vi "PH_ImageCoG_Plotter.Reset.vi"(0 "i ref in":refnum<vi>, 5 "error in":errorcluster) -> (14 "i ref out":refnum<vi>, 19 "error out":errorcluster)   [LabVIEW 2014, in "PH_ImageCoG_Plotter.lvlib"]
doc: "This VI resets some GUI elements and some attributes."
uses:
  PH_ImageCoG_Plotter.lvlib
  <vilib>/vision/Image Controls.llb/IMAQ Image.ctl
  PH_Common/PH_Common.lvlib
  PH_Img_BaseClass/PH_Img_BaseClass.lvlib
panel:
  in  "Image":T1
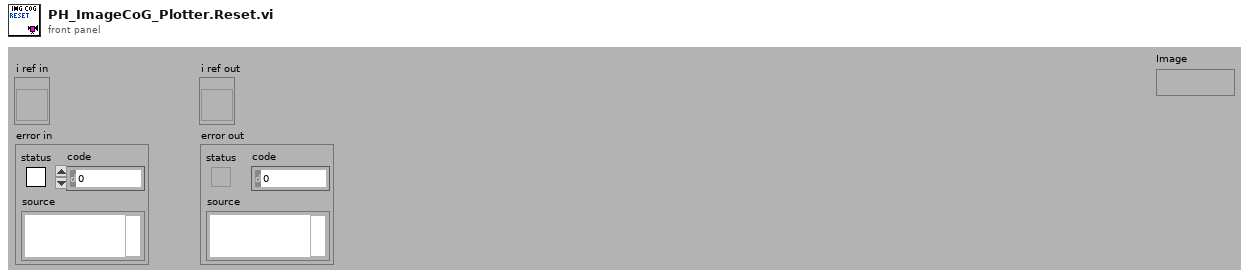
[diagram p1: front panel]
types:
  T1 = typedef "IMAQ Image.ctl" = refnum<image>
  T2 = typedef "PH_ImageCoG_Plotter.lvlib/PH_ImageCoG_Plotter.i attribute.ctl" = cluster{"GUI Refs":cluster{"Delete":refnum<vi>, "Calibration status":refnum<vi>, "BI subtracted":refnum<vi>, "calc Beam Anal":refnum<vi>, "CoG - x":refnum<vi>, "CoG - y":refnum<vi>, "Type":refnum<vi>, "Center":refnum<vi>, "exp - X":refnum<vi>, "exp - Y":refnum<vi>, "Delta - X":refnum<vi>, "Delta - Y":refnum<vi>, "Available Cams":refnum<vi>, "CoG X":refnum<vi>, "CoG Y":refnum<vi>, "Delta X":refnum<vi>, "Delta Y":refnum<vi>, "Export Data":refnum<vi>, "Calibration data":refnum<vi>}, "Calibration":cluster{"Status":T3, "Calibration data":T4, "Calibration Data File":path}, "Beam Analysis":cluster{"on":bool, "exp - X":i32, "exp - Y":i32, "Type":bool, "Data":cluster{"current time":timestamp, "CoG-x":dbl, "CoG-y":dbl, "Delta-x":dbl, "Delta-y":dbl}[], "Datasets strored":i32, "Dataarray Size":i32}, "Cam instances":string[], "DIM Service Events":T5[], "Images":cluster{"Background":T1, "OP":T1, "GUI":T1}}
  T3 = typedef "PH_StatusHandler.lvlib/PH_StatusHandler.Status.ctl" = i16
  T4 = typedef "PH_ImageCalibrator.lvlib/PH_ImageCalibrator.Calibration Data.ctl" = cluster{"Date":string, "Time":string, "Cam Settings":cluster{"Cam ID":string, "Gain":dbl, "Brightness":dbl, "Shutter":dbl, "Cam Error":bool, "Mode":i32}, "Background Image":cluster{"Image":dbl[][], "Image Error":bool}, "Linear Calibration":cluster{"Calibration Factor":dbl, "not mm or mrad":bool}, "Energy Calibration":cluster{"Calibration Factor":dbl, "no mJ":bool}}
  T5 = typedef "BaseProcess.lvlib/BaseProcess.event definition.ctl" = cluster{"CAEEvtDef":T6, "Data Descriptor":T7}
  T6 = typedef "CAEObj.lvlib/CAEObj.event definition.ctl" = cluster{"URL":string, "enable":bool, "ignoreResID":bool}
  T7 = typedef "BaseProcess.lvlib/BaseProcess.descriptor string definition.ctl" = string
  T8 = cluster{"current time":timestamp, "CoG-x":i32, "CoG-y":i32, "Delta-y":dbl, "Delta-x":dbl}[]
  T9 = typedef "PH_Img_BaseClass.lvlib/PH_Img_BaseClass.i attribute.ctl" = cluster{"GUI Refs":T10, "Timeout Image [ms]":i32, "Default Periodic Period [ms]":i32, "Camera":cluster{"Instancename":string, "Notifier":refnum<notifier>}, "Palette":T11, "Cam Settings":cluster{"Cam ID":string, "Gain":dbl, "Brightness":dbl, "Shutter":dbl, "Cam Info Failure":bool, "Mode":i32}}
  T10 = typedef "PH_Img_BaseClass.lvlib/PH_Img_BaseClass.GUI Refs.ctl" = cluster{"Timeout":refnum<vi>, "Image":refnum<vi>, "Palette":refnum<vi>, "Timeout Set":refnum<vi>}
  T11 = typedef "PH_Img_BaseClass.lvlib/PH_Img_BaseClass.Palette.ctl" = i32
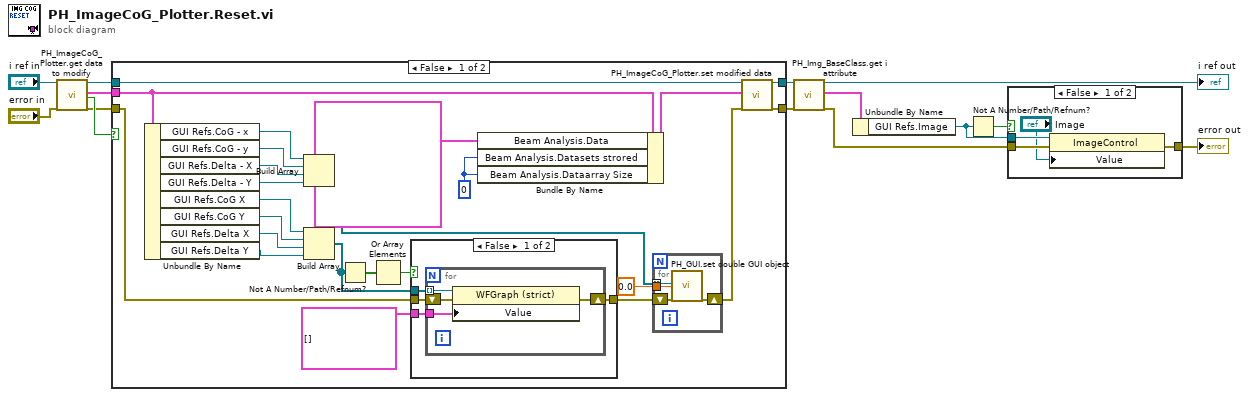
[diagram p0: block diagram]
diagram:
  n1 = call "PH_ImageCoG_Plotter.get data to modify.vi"("i ref in"="i ref in", "error in (no error)"="error in") -> ("i ref out"=w11:refnum<vi>, "i attribute"=w14:T2, "timed out"=w13:bool, "error out"=w12:errorcluster)  [unwired: 14 in]
  n2 = case shown="False" w13 {
    tunnel: w11 -> [w17 w53]
    tunnel: [w35 w53] -> w7
    tunnel: w12 -> [w24 w52]
    tunnel: [w36 w52] -> w8
    tunnel: w14 -> [w37 _]
    frame False {
      w18 = 0
      n3 = Unbundle By Name(w37) -> ("GUI Refs.CoG - x"=w30:refnum<vi>, "GUI Refs.CoG - y"=w31:refnum<vi>, "GUI Refs.Delta - X"=w32:refnum<vi>, "GUI Refs.Delta - Y"=w33:refnum<vi>, "GUI Refs.CoG X"=w25:refnum<vi>, "GUI Refs.CoG Y"=w26:refnum<vi>, "GUI Refs.Delta X"=w27:refnum<vi>, "GUI Refs.Delta Y"=w28:refnum<vi>)
      n4 = Build Array(w30, w31, w32, w33) -> (w15:refnum<vi>[])
      n5 = Build Array(w25, w26, w27, w28) -> (w20:refnum<vi>[])
      n6 = Not A Number/Path/Refnum?(number/path/refnum=w20) -> (NaN/Path/Refnum?=w22:bool[])
      n7 = Or Array Elements(Boolean array=w22) -> (logical OR=w21:bool)
      n8 = case shown="False" w21 {
        tunnel: w24 -> [w42 w47]
        tunnel: [w41 w47] -> w23
        tunnel: w20 -> [w40 _]
        tunnel: cluster{dbl[], dbl[]}[] [] ("Value") -> [w39 _]
        frame False {
          n9 = for {
            tunnel: w40 -> [w44] mode=indexing
            shift-right: [w45] -> w41
            shift-left: w42 -> [w46]
            tunnel: w39 -> [w43]
            n10 = property class="WFGraph (strict)"(reference=w44, error in=w46, "Value"=w43) -> (error out=w45:errorcluster)  [unwired: 1 out]
          }
        }
        frame True {
        }
      }
      n11 = Bundle By Name(cluster=w37, "Beam Analysis.Data"=T8 [], "Beam Analysis.Datasets strored"=w18, "Beam Analysis.Dataarray Size"=w18) -> (w38:T2)
      n12 = for {
        tunnel: w15 -> [w49] mode=indexing
        tunnel: 0.0 ("value") -> [w48]
        shift-right: [w50] -> w16
        shift-left: w23 -> [w51]
        n13 = call "PH_GUI.set double GUI object.vi"("GUI object Ref"=w49, "value"=w48, "error in (no error)"=w51) -> ("error out"=w50:errorcluster)  [unwired: 16 in]
      }
      n14 = call "PH_ImageCoG_Plotter.set modified data.vi"("i ref in"=w17, "i attribute"=w38, "error in (no error)"=w16) -> ("i ref out"=w35:refnum<vi>, "error out"=w36:errorcluster)  [unwired: 15 in]
    }
    frame True {
    }
  }
  n15 = call "PH_Img_BaseClass.get i attribute.vi"("i ref in"=w7, "error in (no error)"=w8) -> ("i ref out"=→"i ref out":refnum<vi>, "i attribute"=w5:T9, "error out"=w2:errorcluster)  [unwired: 15 in]
  n16 = Unbundle By Name(w5) -> ("GUI Refs.Image"=w3:refnum<vi>)
  n17 = Not A Number/Path/Refnum?(number/path/refnum=w3) -> (NaN/Path/Refnum?=w4:bool)
  n18 = case shown="False" w4 {
    tunnel: w2 -> [w57 w58]
    tunnel: [w56 w58] -> w1
    tunnel: w3 -> [w55 _]
    frame False {
      n19 = property class="ImageControl"(reference=w55, error in=w57, "Value"="Image") -> (error out=w56:errorcluster)  [unwired: 1 out]
    }
    frame True {
    }
  }
  "error out" <- w1
